vi "xygraph2.vi"(6 "Chart History (10,000)":i32, 9 "Y Value":dbl, 10 "X Value":dbl, 11 "clear 2":bool) -> (3 "Cluster":cluster{dbl[], dbl[]})   [LabVIEW 2017]
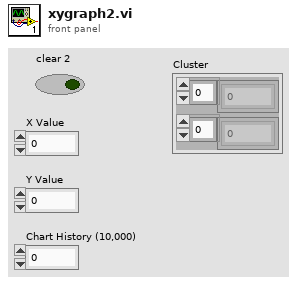
[diagram p1: front panel]
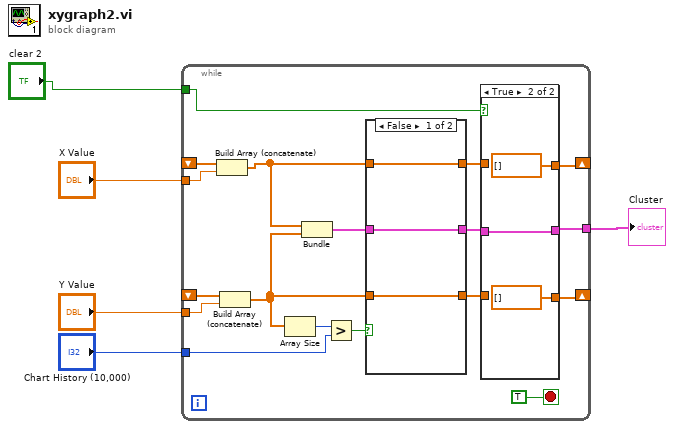
[diagram p0: block diagram]
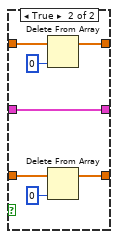
[diagram p3: hidden frame]
diagram:
  n1 = while {
    tunnel: "X Value" -> [w23]
    tunnel: "Y Value" -> [w21]
    shift-right: [w7] -> _
    shift-left: _ -> [w22]
    shift-right: [w10] -> _
    shift-left: _ -> [w20]
    tunnel: "Chart History (10,000)" -> [w18]
    tunnel: [w6] -> w5
    tunnel: "clear 2" -> [w9]
    stop <- TRUE stop-if-true
    n2 = Build Array (concatenate)(w22, w23) -> (w14:dbl[])
    n3 = Build Array (concatenate)(w20, w21) -> (w15:dbl[])
    n4 = Array Size(array=w15) -> (size(s)=w19:i32)
    n5 = Bundle(w14, w15) -> (w16:cluster{dbl[], dbl[]})  [unwired: 1 in]
    n6 = Greater?(x=w19, y=w18) -> (0:w17:bool)
    n7 = case shown="False" w17 {
      tunnel: w16 -> [w30 w33]
      tunnel: w15 -> [w32 w35]
      tunnel: [w32 w34] -> w11
      tunnel: [w31 w38] -> w8
      tunnel: w14 -> [w31 w39]
      tunnel: [w30 w33] -> w12
      frame False {
      }
      frame True {
        n8 = Delete From Array(array=w39, index=0) -> (array with subset deleted=w38:dbl[])  [unwired: 1 in, 1 out]
        n9 = Delete From Array(array=w35, index=0) -> (array with subset deleted=w34:dbl[])  [unwired: 1 in, 1 out]
      }
    }
    n10 = case shown="True" w9 {
      tunnel: [w26 dbl[] []] -> w10
      tunnel: [w25 dbl[] []] -> w7
      tunnel: [w24 w27] -> w6
      tunnel: w12 -> [w24 w27]
      tunnel: w11 -> [w26 _]
      tunnel: w8 -> [w25 _]
      frame False {
      }
      frame True {
      }
    }
  }
  "Cluster" <- w5
